vi "Copy Parse State.vi"(8 "error in (no error)":errorcluster, 10 "From":refnum<class "Packet.lvclass">, 11 "Packet in":refnum<class "Packet.lvclass">) -> (0 "error out":errorcluster, 3 "Packet out":refnum<class "Packet.lvclass">)   [LabVIEW 2020, in "Packet.lvclass"]
uses:
  Packet.lvclass
  Packet.lvclass/Packet.ctl
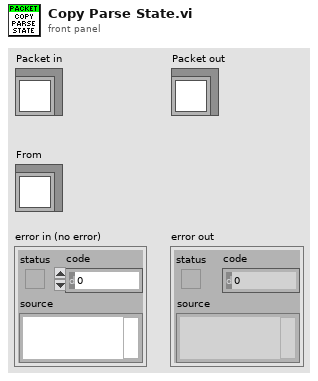
[diagram p1: front panel]
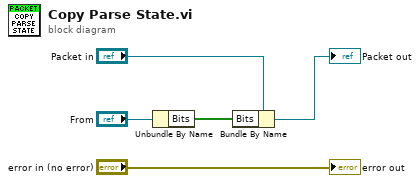
[diagram p0: block diagram]
diagram:
  n1 = Unbundle By Name("From") -> ("Bits"=w3:bool[])
  n2 = Bundle By Name(cluster="Packet in", "Bits"=w3) -> (→"Packet out":refnum<class "Packet.lvclass">)
  "error out" <- "error in (no error)"
